vi "ep_Speed Estimation Peak Search.vi"(0 "spectra points in window":T1(array[cluster]), 5 "frequencies excluded":dbl[](array[numeric]), 7 "pole pairs":i32, 11 "error in (no error)":errorcluster) -> (4 "dup spectra points in window":T1(array[cluster]), 6 "peaks information":T2(array[cluster]), 8 "enough points for peak search?":bool[](array[boolean]), 10 "number of peaks":i32[](array[numeric]), 14 "minimum max-magnitude":dbl, 15 "error out":errorcluster)   [LabVIEW 2014, in "NI_EP_Motor Monitoring.lvlib"]
uses:
  <vilib>/addons/Electrical Power/Motor Monitoring/NI_EP_Motor Monitoring.lvlib
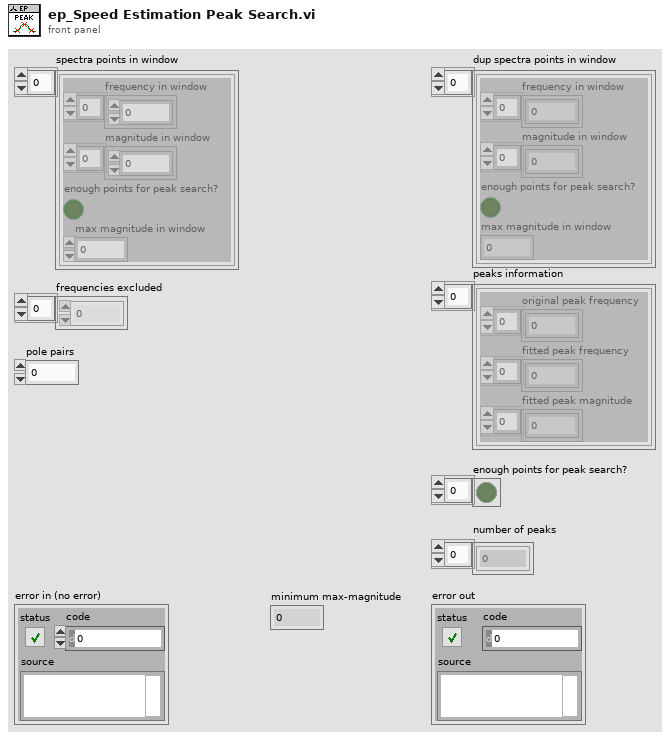
[diagram p1: front panel]
types:
  T1 = cluster{"frequency in window":dbl[], "magnitude in window":dbl[], "enough points for peak search?":bool, "max magnitude in window":dbl}[]
  T2 = cluster{"original peak frequency":dbl[], "fitted peak frequency":dbl[], "fitted peak magnitude":dbl[]}[]
  T3 = cluster{"peak frequency":dbl[], "fitted peak frequency":dbl[], "fitted peak magnitude":dbl[]}
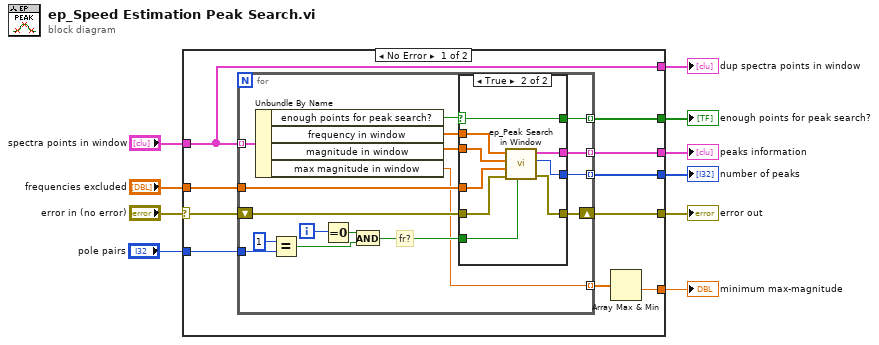
[diagram p0: block diagram]
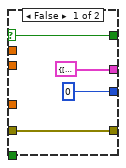
[diagram p2: hidden frame]
diagram:
  n1 = case shown="No Error" "error in (no error)" {
    selector: "error in (no error)" -> [w20 w51]
    tunnel: [w17 w51] -> w9
    tunnel: "frequencies excluded" -> [w19 _]
    tunnel: [w18 _] -> w7
    tunnel: "spectra points in window" -> [w16 _]
    tunnel: [w16 _] -> w6
    tunnel: "pole pairs" -> [w15 _]
    tunnel: [w13 _] -> w3
    tunnel: [w12 _] -> w2
    tunnel: [w11 _] -> w1
    frame No Error {
      n2 = for {
        tunnel: w19 -> [w36]
        tunnel: [w35] -> w18 mode=indexing
        tunnel: [w33] -> w12 mode=indexing
        shift-right: [w34] -> w17
        shift-left: w20 -> [w37]
        tunnel: w16 -> [w32] mode=indexing
        tunnel: [w28] -> w11 mode=indexing
        tunnel: w15 -> [w26]
        tunnel: [w21] -> w14 mode=indexing
        i -> [w27]
        # "fr?"
        n3 = Unbundle By Name(w32) -> ("enough points for peak search?"=w31:bool, "frequency in window"=w30:dbl[], "magnitude in window"=w29:dbl[], "max magnitude in window"=w21:dbl)
        n4 = Equal?(x=1, y=w26) -> (x = y?=w23:bool)
        n5 = Equal To 0?(x=w27) -> (x = 0?=w24:bool)
        n6 = And(x=w24, y=w23) -> (x .and. y?=w22:bool)
        n7 = case shown="True" w31 {
          selector: w31 -> [w38 w43]
          tunnel: w37 -> [w41 w50]
          tunnel: w36 -> [_ w46]
          tunnel: [T3 {"peak frequency"=[], "fitted peak frequency"=[], "fitted peak magnitude"=[]} ("peaks information") w49] -> w35
          tunnel: [w41 w48] -> w34
          tunnel: [0 ("number of peaks") w47] -> w33
          tunnel: w30 -> [_ w45]
          tunnel: w29 -> [_ w44]
          tunnel: [w38 w43] -> w28
          tunnel: w22 -> [_ w42]
          frame False {
          }
          frame True {
            n8 = call <vilib>:"ep_Peak Search in Window.vi"("fr when 1 polepairs? (F)"=w42, "error in (no error)"=w50, "frequency excluded"=w46, "magnitude in window"=w44, "frequency in window"=w45) -> ("error out"=w48:errorcluster, "number of peaks"=w47:i32, "peaks information"=w49:T3)  [unwired: 4 in]
          }
        }
      }
      n9 = Array Max & Min(array=w14) -> (min value=w13:dbl)  [unwired: 3 out]
    }
    frame Error {
    }
  }
  "error out" <- w9
  "dup spectra points in window" <- w6
  "peaks information" <- w7
  "minimum max-magnitude" <- w3
  "number of peaks" <- w2
  "enough points for peak search?" <- w1
